vi "acknowledgeIRQs.vi"(8 "error in (no error)":errorcluster, 10 "IRQs":i32[](array[numeric]), 11 "ModbusIRQs in":refnum<class "ModbusIRQs.lvclass">) -> (0 "error out":errorcluster, 3 "ModbusIRQs out":refnum<class "ModbusIRQs.lvclass">)   [LabVIEW 2016, in "ModbusIRQs.lvclass"]
uses:
  ModbusIRQs.lvclass
  ModbusIRQs.lvclass/ModbusIRQs.ctl
  <vilib>/Utility/error.llb/Error Cluster From Error Code.vi
  <vilib>/rvi/interface/nirviMethod/nirviMethod.xnode
  <vilib>/FPGAPlugInAG/Dynamic/niLvFpga_AcknowledgeIrq_Dynamic.vi
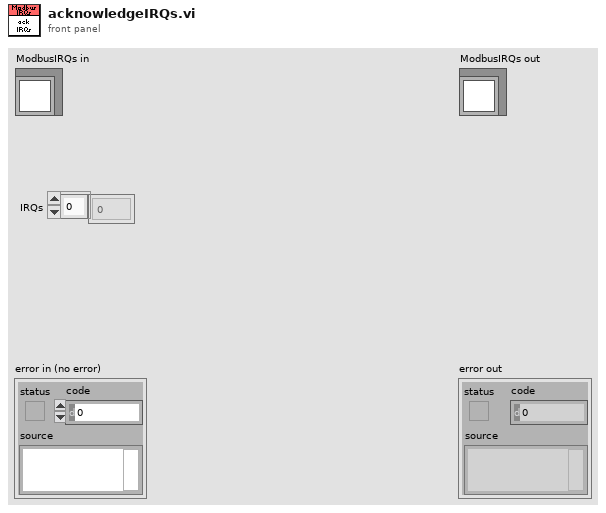
[diagram p1: front panel]
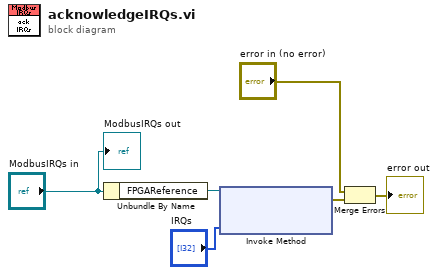
[diagram p0: block diagram]
diagram:
  n1 = Unbundle By Name("ModbusIRQs in") -> ("FPGAReference"=w6:refnum<k20>)
  n2 = xnode "Invoke Method"("FPGA VI Reference In"=w6, "IRQ Number(s)"="IRQs") -> ("error out"=w1:errorcluster)  [unwired: 1 in, 1 out]
  n3 = Merge Errors("error in (no error)", w1) -> (→"error out":errorcluster)
  "ModbusIRQs out" <- "ModbusIRQs in"
